vi "Falcon2Config.vi"() -> (3 "IMAQ Camera serial config":T1)   [LabVIEW 2011]
uses:
  GenericIMAQCamera/GenericIMAQHardwareConfig.ctl
panel:
  in  "IMAQ Camera serial config 2":T1={"Use serial commands directly"=TRUE, "Frame rate set cmd"="ssf %d", "Exposure time set cmd"="set %d", "Frame rate get cmd"="get ssf", "Exposure time get cmd"="get set", "IMAQ Identifier"="img0", "Serial return skip chars"=1, "Set width/height"="aiw %d\raih %d", "Set offset xy"="aix %d\raiy %d", "Get width"="get aiw", "Get height"="get aih", "Get offset X"="get aix", "Get offset Y"="get aiy", "Full frame size"={"width"=4096, "height"=3072}}
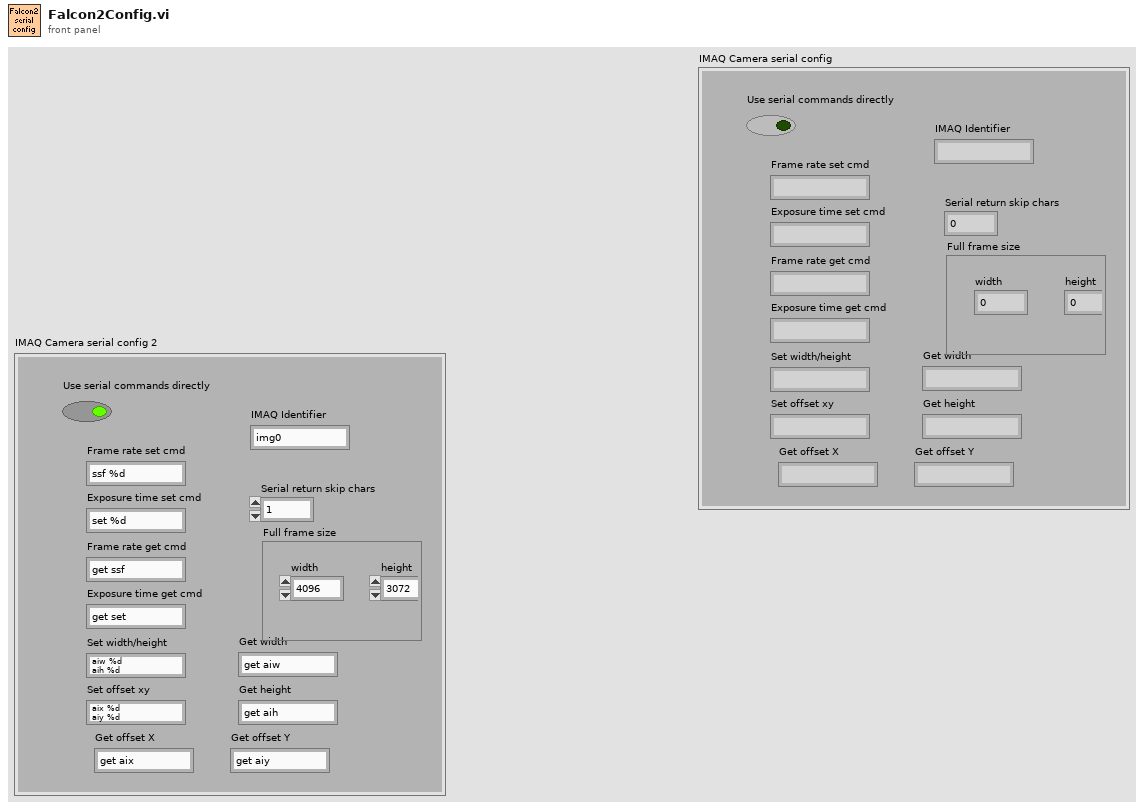
[diagram p1: front panel]
types:
  T1 = typedef "GenericIMAQHardwareConfig.ctl" = cluster{"Use serial commands directly":bool, "Frame rate set cmd":string, "Exposure time set cmd":string, "Frame rate get cmd":string, "Exposure time get cmd":string, "IMAQ Identifier":string, "Serial return skip chars":i32, "Set width/height":string, "Set offset xy":string, "Get width":string, "Get height":string, "Get offset X":string, "Get offset Y":string, "Full frame size":cluster{"width":i32, "height":i32}}
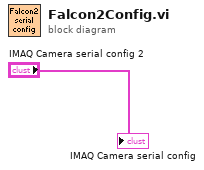
[diagram p0: block diagram]
diagram:
  "IMAQ Camera serial config" <- "IMAQ Camera serial config 2"
